vi "ui--test the theme.vi"() -> ()   [LabVIEW 2021]
doc: "a test interface to understand what it will look like when a theme is used on a program\n\n<b>Code Developed By:</b> +\nDaniel Coons +\nTechnology Service Corporation +\nwww.tsc.com/atcs"
panel:
  in  "Tab Control":T1(tab)
  in  "Selector Button":bool caption="Part Number"
  in  "File Path":path=path "C:/path"
  in  "String":string="text is here"
  in  "Enum":enum16{"Choice 1"}(ring)
  in  "Text Ring":u16(ring) items=["Choice 1"]
  in  "Combo Box":string(combo)="Choice 1"
  in  "DAQmx Task Name":refnum<k21>="PCI-6221/ai0"
  in  "Digital Numeric":dbl caption="Numeric"
  out "LED":bool
  in  "Color Box":u32(colorbox)
  in  "Cluster":cluster{"Numeric":dbl, "String":string}
  in  "Array - Numeric":dbl[](array[numeric])
  in  "Horizontal Pointer Slide":dbl(slide) scale=0.0..10.0
  in  "Horizontal Slide":dbl(slide)=3.697478991596639 scale=0.0..10.0
  in  "Table":i32(listbox)=-1 caption="Datasheets"
  in  "listbox":i32(listbox)=3 caption="parts-listbox"
  in  "Tree":string(tree)="item"
  in  "Tree 2":string(tree)="top item"
  in  "Table Control":string[][](table)=[["val 0,0"]]
  in  "Multicolumn Listbox":i32(listbox)
  in  "elevated--rectangular--icon":bool
  in  "elevated--rounded--icon":bool
  in  "filled--rectangular--icon":bool
  in  "filled--rounded--icon":bool
  in  "nooutline--rectangular--icon":bool
  in  "nooutline--rounded--icon":bool
  in  "outline--rectangular--icon":bool
  in  "outline--rounded--icon":bool
  in  "tonal--rectangular--icon":bool
  in  "tonal--rounded--icon":bool
  in  "transparent--rectangular--icon":bool
  in  "transparent--rounded--icon":bool
  in  "elevated--rectangular--icon--mulitple--large":bool
  in  "FAB--rounded--icon--large":bool
  in  "elevated--rectangular--icon 2":bool caption="elevated--rectangular--icon"
  in  "elevated--rounded--icon 2":bool caption="elevated--rounded--icon"
  in  "filled--rectangular--icon 2":bool caption="filled--rectangular--icon"
  in  "filled--rounded--icon 2":bool caption="filled--rounded--icon"
  in  "nooutline--rectangular--icon 2":bool caption="nooutline--rectangular--icon"
  in  "nooutline--rounded--icon 2":bool caption="nooutline--rounded--icon"
  in  "outline--rectangular--icon 2":bool caption="outline--rectangular--icon"
  in  "outline--rounded--icon 2":bool caption="outline--rounded--icon"
  in  "tonal--rectangular--icon 2":bool caption="tonal--rectangular--icon"
  in  "tonal--rounded--icon 2":bool caption="tonal--rounded--icon"
  in  "transparent--rectangular--icon 2":bool caption="transparent--rectangular--icon"
  in  "transparent--rounded--icon 2":bool caption="transparent--rounded--icon"
  in  "elevated--rectangular--icon--mulitple--large 2":bool caption="elevated--rectangular--icon--mulitple--large"
  in  "FAB--rounded--icon--large 2":bool caption="FAB--rounded--icon--large"
  in  "elevated--rectangular--icon 3":bool caption="elevated--rectangular--icon"
  in  "elevated--rounded--icon 3":bool caption="elevated--rounded--icon"
  in  "filled--rectangular--icon 3":bool caption="filled--rectangular--icon"
  in  "filled--rounded--icon 3":bool caption="filled--rounded--icon"
  in  "nooutline--rectangular--icon 3":bool caption="nooutline--rectangular--icon"
  in  "nooutline--rounded--icon 3":bool caption="nooutline--rounded--icon"
  in  "outline--rectangular--icon 3":bool caption="outline--rectangular--icon"
  in  "outline--rounded--icon 3":bool caption="outline--rounded--icon"
  in  "tonal--rectangular--icon 3":bool caption="tonal--rectangular--icon"
  in  "tonal--rounded--icon 3":bool caption="tonal--rounded--icon"
  in  "transparent--rectangular--icon 3":bool caption="transparent--rectangular--icon"
  in  "transparent--rounded--icon 3":bool caption="transparent--rounded--icon"
  in  "elevated--rectangular--icon--mulitple--large 3":bool caption="elevated--rectangular--icon--mulitple--large"
  in  "FAB--rounded--icon--large 3":bool caption="FAB--rounded--icon--large"
  in  "filled--rectangular--icon--multiple--large (false) 2":bool
  in  "filled--rectangular--icon--multiple--large (true) 2":bool
  in  "elevated--rectangular--icon--multiple (false) 2":bool
  in  "elevated--rectangular--icon--multiple (true) 2":bool
  in  "filled--rectangular--icon--multiple--large (false)":bool
  in  "filled--rectangular--icon--multiple--large (true)":bool
  in  "elevated--rectangular--icon--multiple (false)":bool
  in  "elevated--rectangular--icon--multiple (true)":bool
  out "Waveform Chart":T2(graph)={"number: 0 to 1"=0.9587742130972315, "number: 0 to 1"=2.621710596199856, "number: 0 to 1"=4.648407460731506, "number: 0 to 1"=6.613308533487236}
  out "Waveform Graph":dbl[][](graph)=[[0.8166996489636194, 0.7544537833390327, 0.9763419481683275, 0.581441397966104, 0.7059064313545167, 0.7222064659111673, 0.21543216864216852, 0.5141296914745976, 0.8256485708247667, 0.5334188869476608, 0.1225197602369259, 0.161102845321484, 0.7388459282410049, 0.46613893443934185, 0.7574774420510761, 0.14136303803810657, 0.4008209964368885, 0.4821014561002759, 0.34330959643655246, 0.2289152428543888, 0.19366060017910353, 0.15952083905471115, 0.9099031814170742, 0.04060803447488315, 0.881148534257798, 0.11441049681183446, 0.37755849607722736, 0.28713752122816216, 0.1756345478876984, 0.4056118685520156, 0.15672042202388337, 0.07806378520624424, 0.7850958512929871, 0.2217421490387408, 0.6240379616240912, 0.12697532393283772, 0.8951512543314877, 0.45286635629869787, 0.5607854594121331, 0.4181410551127154, 0.18043846138947606, 0.12377313755693753, 0.07411534005405063, 0.918482514153526, 0.2743797292156942, 0.2985783667453197, 0.3421640772537613, 0.2599516360312839, 0.8148656978795061, 0.6215189723113068, 0.7687052698452588, 0.5425397831633332, 0.6815428220989486, 0.05404617095239539, 0.043653527391962044, 0.7282588924926658, 0.23869078674262, 0.5049072640965286, 0.177050874331661, 0.8334220264149867, 0.8054746361885083, 0.21518046712046912, 0.010499894012597544, 0.7254368753187632, 0.02023549591166418, 0.49729143861074765, 0.40640447258793877, 0.3748947832594389, 0.7925907351920509, 0.6979886660586314, 0.33580169472202215, 0.6840950584259766, 0.9943403660516035, 0.815570440575653, 0.5179774565079667, 0.8561196695833952, 0.9966465918548373, 0.7516845203147005, 0.374531991012784, 0.6905582027378565, 0.2299966956734094, 0.7779878702029315, 0.9736569437180416, 0.5122970593859255, 0.14450409568110079, 0.07282558806510586, 0.9600573428913353, 0.3617499859322657, 0.2808587214377929, 0.7650085392273682, 0.36027942253099665, 0.585803476479043, 0.3821585791046842, 0.7186192706576495, 0.7513439002920002, 0.9016268040199902, 0.24298812111916046, 0.701619904408364, 0.6122222576914085, 0.8938843318835699], [2.305426048223438, 2.7282095691655504, 2.368548485865656, 2.523706026559939, 2.8251250354383277, 2.920349002618986, 2.601720379611918, 2.009540053771827, 2.6059623023821974, 2.952938925756414, 2.28304062782485, 2.2417999525154366, 2.899760688737934, 2.8625481266476247, 2.114626784333246, 2.790891797990594, 2.57188027723174, 2.271016491819438, 2.175405867936157, 2.1358846561500986, 2.055038372441022, 2.5167937671642147, 2.755232022680961, 2.3149244647757605, 2.600328568904907, 2.487342501826031, 2.9048393537298773, 2.3813105710759586, 2.2973652973438354, 2.1847051474996126, 2.382929707542842, 2.119322078584429, 2.978125204670463, 2.4617549244026073, 2.946877403545415, 2.8309900755221715, 2.410524944884685, 2.3807149863981385, 2.854786726712487, 2.5709752054318775, 2.469629863103202, 2.658180379425045, 2.6418511113151673, 2.471086715529773, 2.428638680169859, 2.4534035125743734, 2.974817574617668, 2.1648822294074392, 2.3363154459519015, 2.5966870170566745, 2.579216331134022, 2.2418449724707195, 2.0042351927073367, 2.8723021392904053, 2.5075752784416787, 2.430799399297558, 2.0700539756564065, 2.0480038630359196, 2.579592968927077, 2.0167608806963484, 2.7792456949627655, 2.483419212939858, 2.0771196836975734, 2.706841852172321, 2.9184446525674197, 2.0844257212347252, 2.043118166505069, 2.1271244642462044, 2.7862504755942332, 2.291493378837396, 2.4780928561199915, 2.707447003748201, 2.21271049812406, 2.8587369399518514, 2.458354912865303, 2.013264068854178, 2.044037806670537, 2.9392698231289325, 2.6357761558243133, 2.320608372639952, 2.602591531237705, 2.9319586019400967, 2.247994225443691, 2.708408037128834, 2.151923236811828, 2.013774941266835, 2.5783309184814143, 2.5793519825392246, 2.1200678408530527, 2.4058338625657463, 2.6884116097316704, 2.6040426972674826, 2.5768580516537707, 2.679813540211224, 2.250384260671651, 2.176342233798596, 2.149049028970377, 2.687447262806155, 2.0042088127141398, 2.0171460835318338], [4.309736497148739, 4.816899228748792, 4.51378905222781, 4.4148430726876065, 4.030969866863546, 4.836220537663333, 4.19963575737237, 4.048251034005039, 4.44201039736347, 4.8464209995966945, 4.277961830964641, 4.5187259048613395, 4.593476769199926, 4.053052799773547, 4.520281417515909, 4.591735849204716, 4.554963037579354, 4.342710583351511, 4.258404273735749, 4.690017938217111, 4.8646825486026914, 4.533420846315398, 4.25416871872749, 4.97538762820963, 4.753919898983899, 4.567772573066251, 4.062504592455236, 4.570916864282702, 4.428726196944439, 4.42983030503869, 4.941586203690884, 4.593473963342996, 4.34558867597536, 4.245880965053614, 4.962774676476811, 4.936816439960061, 4.7271704736253986, 4.52007790716265, 4.624136907831092, 4.36300753429124, 4.023965865194311, 4.052197524326224, 4.635460977983546, 4.4048589236798446, 4.4942492669576275, 4.823727752757078, 4.850897275873713, 4.569133984113497, 4.267795157833008, 4.222821165334924, 4.466349239994772, 4.419865959245668, 4.042727504457708, 4.291476295430478, 4.976060229277514, 4.066698584664963, 4.397145456518063, 4.991171954177278, 4.668744018098164, 4.647925523049323, 4.240802274738044, 4.049085550957804, 4.056010606317652, 4.856521133893583, 4.751145348447303, 4.862668851852531, 4.507177776994613, 4.933227846154707, 4.862948285216264, 4.251434079517253, 4.996094430668099, 4.64013224968455, 4.4471464643084975, 4.7020470815859206, 4.421723521195897, 4.577476552410164, 4.304557903422648, 4.314994262924884, 4.024765754351593, 4.477529059986332, 4.3852994781736925, 4.616820323720316, 4.589095774733753, 4.296542632700815, 4.758233911625293, 4.098670635176005, 4.8480496339612, 4.351486242037636, 4.825157254515511, 4.321338897687887, 4.671811766304071, 4.427520870996878, 4.9884384359046665, 4.787063037055932, 4.42268281043168, 4.809605900878463, 4.414131606373238, 4.16014802640343, 4.591791621881006, 4.681060308635081], [6.6579401345550195, 6.699063573109737, 6.411842951258533, 6.011054140266885, 6.811495267376232, 6.835790388162222, 6.916124384028534, 6.564070494565899, 6.477374598938039, 6.066362979038183, 6.8252894845038465, 6.969932515355096, 6.080930806518948, 6.5314903781335385, 6.6164306225240415, 6.099785725860528, 6.8132911278009205, 6.58474973267365, 6.073031582965795, 6.2198021786044695, 6.335354256884886, 6.3861145323321, 6.815742121217646, 6.435297654777207, 6.883581240684199, 6.332077185393913, 6.527793035369571, 6.8296406446380065, 6.755058989117485, 6.897201755187986, 6.388672866697133, 6.204759003126279, 6.544166333272917, 6.168457058586981, 6.26537521019533, 6.18040737892451, 6.336013881019837, 6.345012003564636, 6.292404713796964, 6.706295905385718, 6.821799088555453, 6.158693554789245, 6.328912153347883, 6.130662251789268, 6.319507600126026, 6.876572954530628, 6.321663826294273, 6.061759686994103, 6.524120564279607, 6.1886113951770625, 6.7588639863751006, 6.714637895521955, 6.062968722335364, 6.123918541009844, 6.89107643014135, 6.87037990716791, 6.160078376823507, 6.447754679889853, 6.653814910386323, 6.758272336582555, 6.3517762178219135, 6.999818077650774, 6.4071002996722575, 6.961204331200356, 6.82631103052828, 6.913590377555749, 6.11981871179368, 6.696981824985835, 6.246034098842474, 6.927558169696511, 6.23832457208741, 6.338319686209528, 6.200695718321706, 6.270809759666021, 6.459439176735021, 6.337997502755655, 6.09997785230265, 6.732943673260452, 6.776623075187863, 6.38335915886811, 6.417896059221185, 6.789406473049253, 6.416120578873585, 6.167176427924493, 6.7735927598645205, 6.341666495133849, 6.997510748803348, 6.797761000162448, 6.7558156035744386, 6.187395078601895, 6.388550812642949, 6.905978107884507, 6.2011953013841214, 6.606857015318475, 6.8419676882750124, 6.77305898157141, 6.840579671613506, 6.057472723052808, 6.983769958492456, 6.033031461754228]]
  out "error out":errorcluster
  in  "error in (no error)":errorcluster
  in  "Close":bool
  in  "Settings":bool
  in  "Tab Control":enum32{"Page 1"}(tab)
  in  "Refresh":bool
  in  "Print":bool
  in  "export":bool
  in  "refresh-continual":bool
  in  "app-settings":bool
  in  "theme":bool
  in  "open":bool
  out "Header":bool
  # "Free Label Text"
  # "Decoration"
  # "Primary"
  # "Secondary"
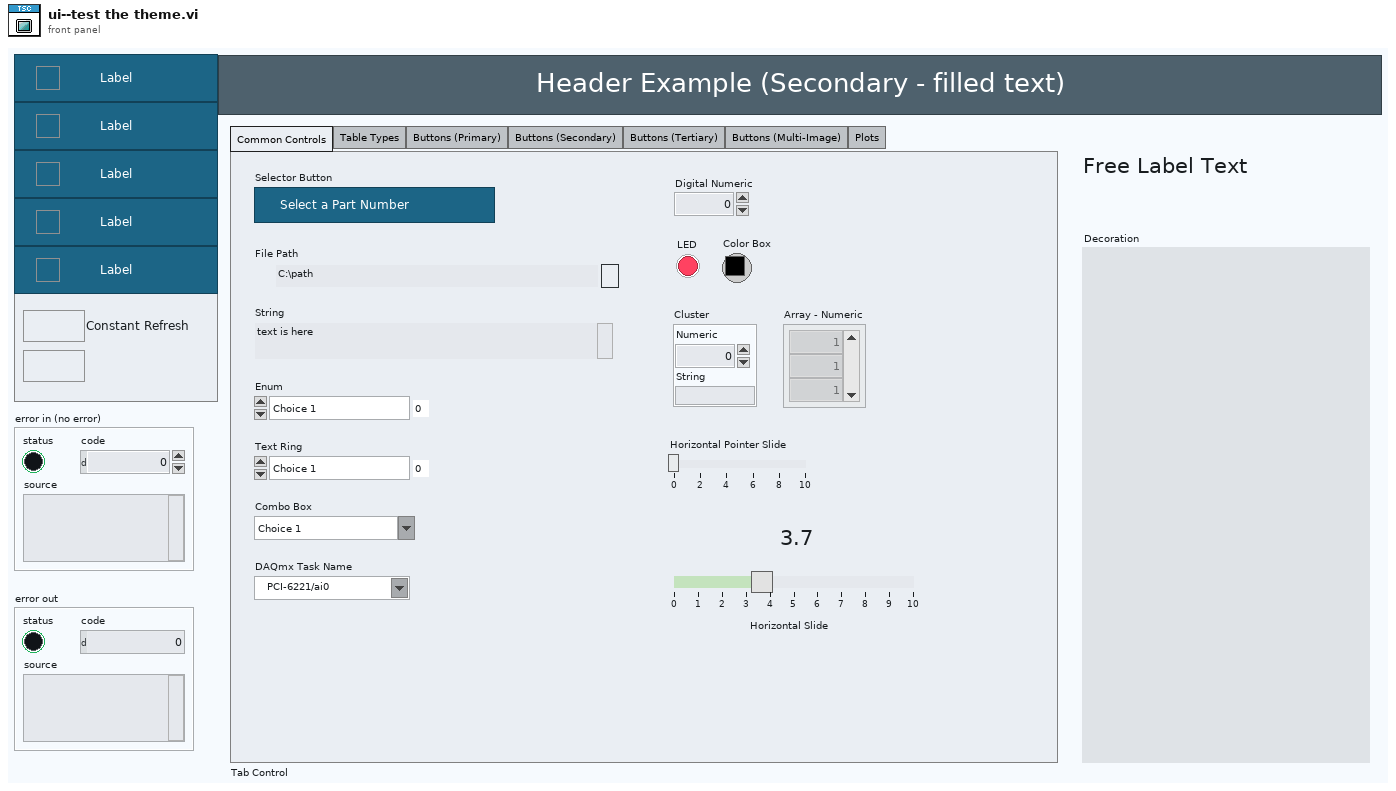
[diagram p1: front panel]
types:
  T1 = enum32{"Common Controls", "Table Types", "Buttons (Primary)", "Buttons (Secondary)", "Buttons (Tertiary)", "Buttons (Multi-Image)", "Plots"}
  T2 = cluster{"number: 0 to 1":dbl, "number: 0 to 1":dbl, "number: 0 to 1":dbl, "number: 0 to 1":dbl}
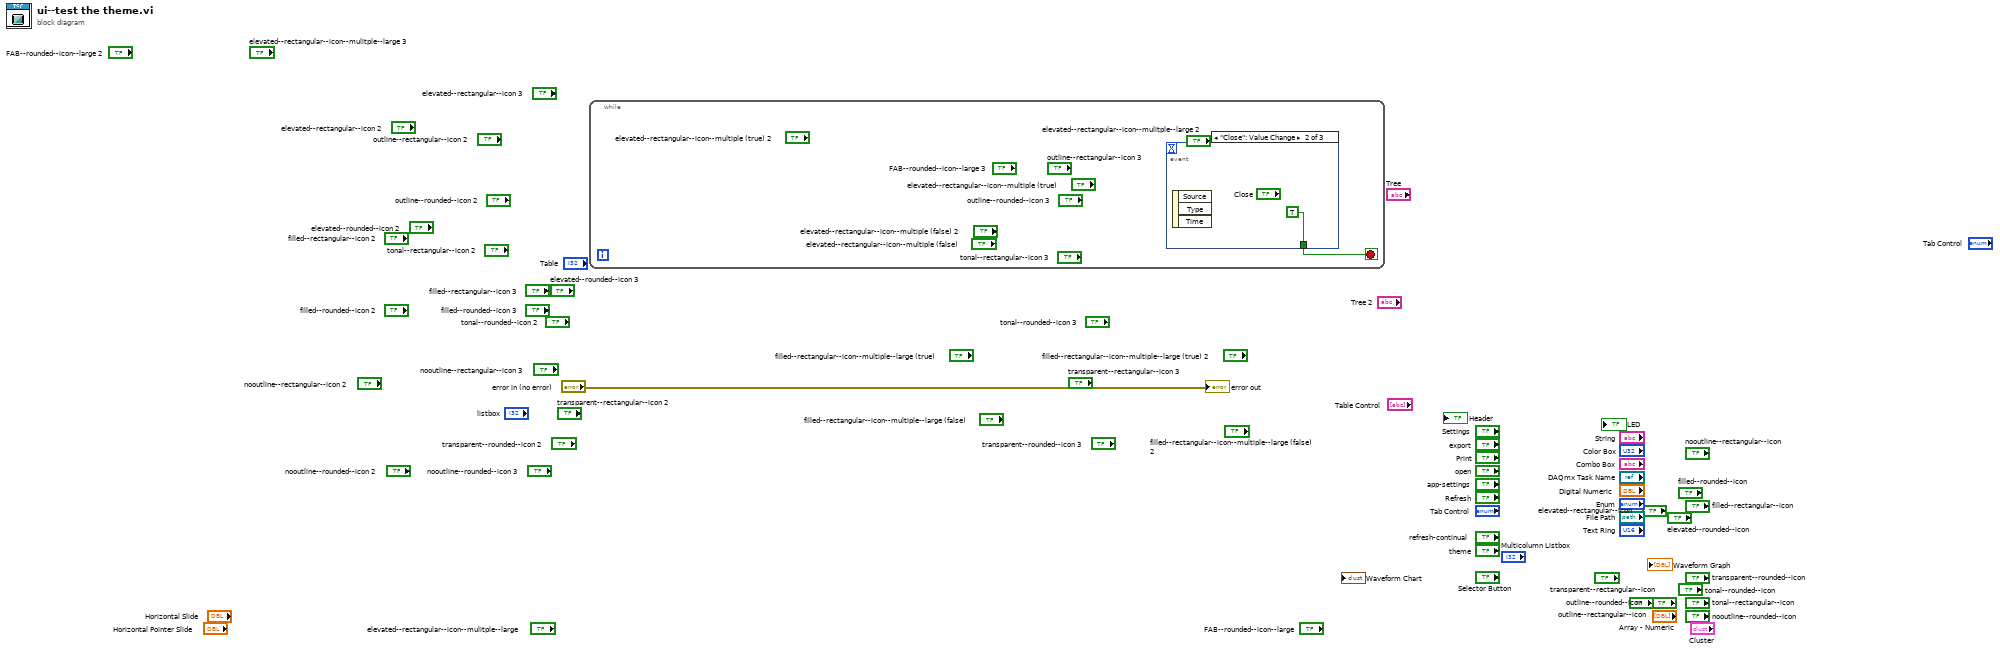
[diagram p0: block diagram]
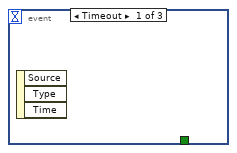
[diagram p2: hidden frame]
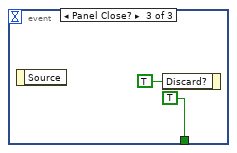
[diagram p3: hidden frame]
diagram:
  n1 = while {
    stop <- w2 stop-if-true
    n2 = event shown="[1] \"Close\": Value Change" {
      selector: _ -> [_ _ _]
      dyn-events: _ -> [_ _ _]
      timeout: _ -> [_ _ _]
      tunnel: [_ TRUE TRUE] -> w2
      event Timeout {
        n3 = event-data() -> ()  [unwired: 1 in, 3 out]
      }
      event "Close": Value Change {
        n4 = event-data() -> ()  [unwired: 1 in, 3 out]
      }
      event Panel Close? {
        n5 = event-data() -> ()  [unwired: 1 in, 1 out]
        n6 = event-data("Discard?"=TRUE) -> ()  [unwired: 1 in, 1 out]
      }
    }
  }
  "error out" <- "error in (no error)"
